vi "Wait for GFG Flag.vi"(7 "Wait for GFG Flag_Command":T1, 8 "error in (no error)":errorcluster, 11 "Listening Variable":string) -> (0 "error out":errorcluster)   [LabVIEW 2012]
doc: "SciScan 1.2 160622"
uses:
  Wait for GFG Flag_Command.ctl
panel:
  out "ms to flag":i32
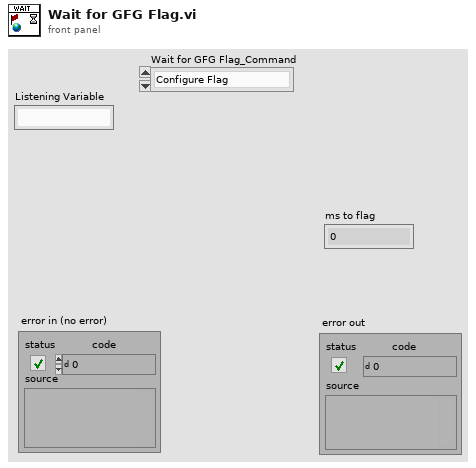
[diagram p1: front panel]
types:
  T1 = typedef "Wait for GFG Flag_Command.ctl" = enum16{"Configure Flag", "Wait for Flag or Exit"}
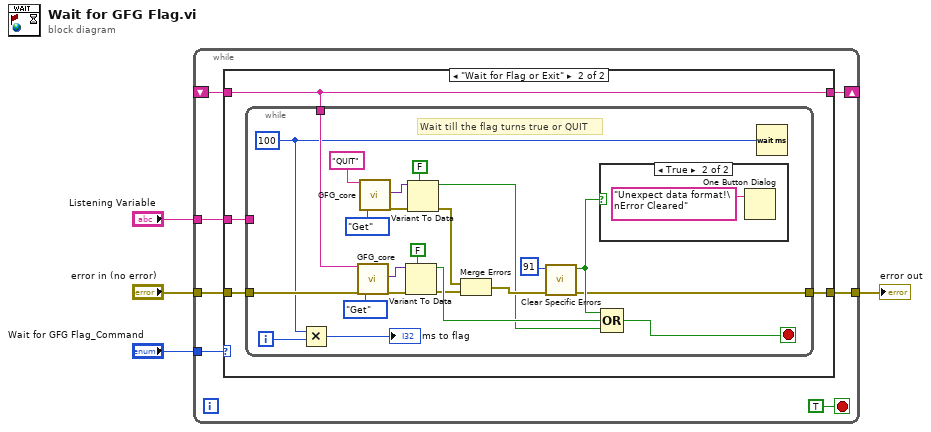
[diagram p0: block diagram]
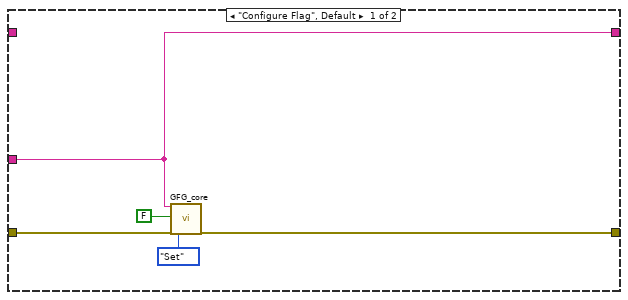
[diagram p2: hidden frame]
diagram:
  n1 = while {
    tunnel: "Listening Variable" -> [w8]
    tunnel: "Wait for GFG Flag_Command" -> [w10]
    shift-right: [w9] -> _
    shift-left: _ -> [w7]
    tunnel: "error in (no error)" -> [w6]
    tunnel: [w5] -> w1
    stop <- TRUE stop-if-true
    n2 = case shown="\"Wait for Flag or Exit\"" w10 {
      tunnel: [w13 w18] -> w9
      tunnel: w8 -> [w13 w20]
      tunnel: w7 -> [_ w18]
      tunnel: w6 -> [w15 w19]
      tunnel: [w12 w17] -> w5
      frame "Configure Flag", Default {
        n3 = call "GFG_core.vi"("Variable Name in"=w13, "Variant in"=FALSE, "error in (no error)"=w15, "Action"=enum16{"Init", "Set", "Get", "Clear"}."Set") -> ("error out"=w12:errorcluster)  [unwired: 9 in, 6 out]
      }
      frame "Wait for Flag or Exit" {
        n4 = while {
          tunnel: w20 -> [_]
          tunnel: w19 -> [w41]
          tunnel: w18 -> [w43]
          tunnel: [w28] -> w17
          i -> [w22]
          stop <- w34 stop-if-true
          w21 = u32 100 ("milliseconds to wait")
          # "Wait till the flag turns true or QUIT"
          n5 = Multiply(x=w21, y=w22) -> (x*y=→"ms to flag":u32)
          n6 = call "GFG_core.vi"("Variable Name in"=w43, "error in (no error)"=w41, "Action"=enum16{"Init", "Set", "Get", "Clear"}."Get") -> ("Variant Out"=w37:variant, "error out"=w39:errorcluster)  [unwired: 10 in, 5 out]
          n7 = call "GFG_core.vi"("Variable Name in"="QUIT" ("Variable Name"), "Action"=enum16{"Init", "Set", "Get", "Clear"}."Get") -> ("Variant Out"=w29:variant, "error out"=w30:errorcluster)  [unwired: 11 in, 5 out]
          n8 = Variant To Data(error in=w39, type=FALSE, Variant=w37) -> (data=w35:bool, error out=w26:errorcluster)
          n9 = Variant To Data(error in=w30, type=FALSE, Variant=w29) -> (data=w24:bool, error out=w27:errorcluster)
          n10 = Merge Errors(w27, w26) -> (w25:errorcluster)
          n11 = call "Clear Specific Errors.vi"("Error In"=w25, "Error number In"=91) -> ("Error Out"=w28:errorcluster, "Error Cleared?"=w36:bool)  [unwired: 8 in]
          n12 = case shown="True" w36 {
            frame False {
            }
            frame True {
              n13 = One Button Dialog(message="Unexpect data format!\nError Cleared") -> ()  [unwired: 1 in, 1 out]
            }
          }
          n14 = Compound Arithmetic op=OR(w36, w35, w24) -> (w34:bool)
          n15 = Wait (ms)(milliseconds to wait=w21) -> ()  [unwired: 1 out]
        }
      }
    }
  }
  "error out" <- w1
